vi "RPC Method queryserver_QueryServer_Register.vi"(8 "error in (no error)":errorcluster, 11 "OOP Server in":refnum<class "TestDataMarshal.lvclass">) -> (0 "error out":errorcluster, 3 "OOP Server out":refnum<class "TestDataMarshal.lvclass">)   [LabVIEW 2019, in "TestDataMarshal.lvlib" / "TestDataMarshal.lvclass"]
uses:
  TestDataMarshal.lvclass
  TestDataMarshal.lvclass/TestDataMarshal.ctl
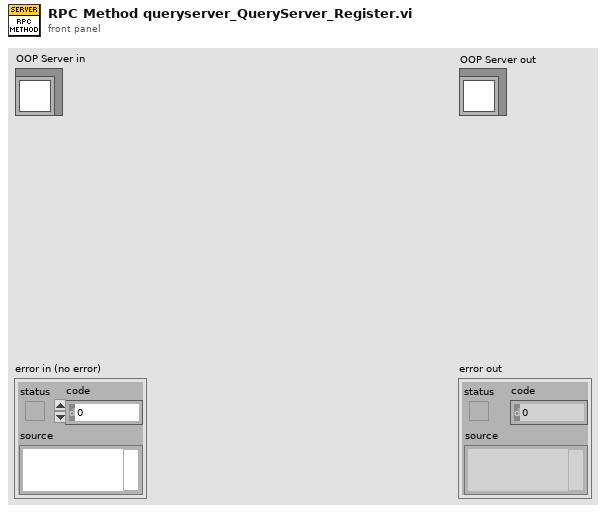
[diagram p1: front panel]
types:
  T1 = typedef "TestDataMarshal.lvlib/TestDataMarshal.lvclass/Server Internal UEs.ctl" = cluster{"queryserver_QueryServer_Invoke Internal UE":refnum<user-event>, "queryserver_QueryServer_Query Internal UE":refnum<user-event>, "queryserver_QueryServer_Register Internal UE":refnum<user-event>, "queryserver_QueryServer_TestDataTypes Internal UE":refnum<user-event>}
  T2 = typedef "TestDataMarshal.lvlib/TestDataMarshal.lvclass/Server gRPC UEs.ctl" = cluster{"queryserver_QueryServer_Invoke gRPC UE":refnum<user-event>, "queryserver_QueryServer_Query gRPC UE":refnum<user-event>, "queryserver_QueryServer_Register gRPC UE":refnum<user-event>, "queryserver_QueryServer_TestDataTypes gRPC UE":refnum<user-event>}
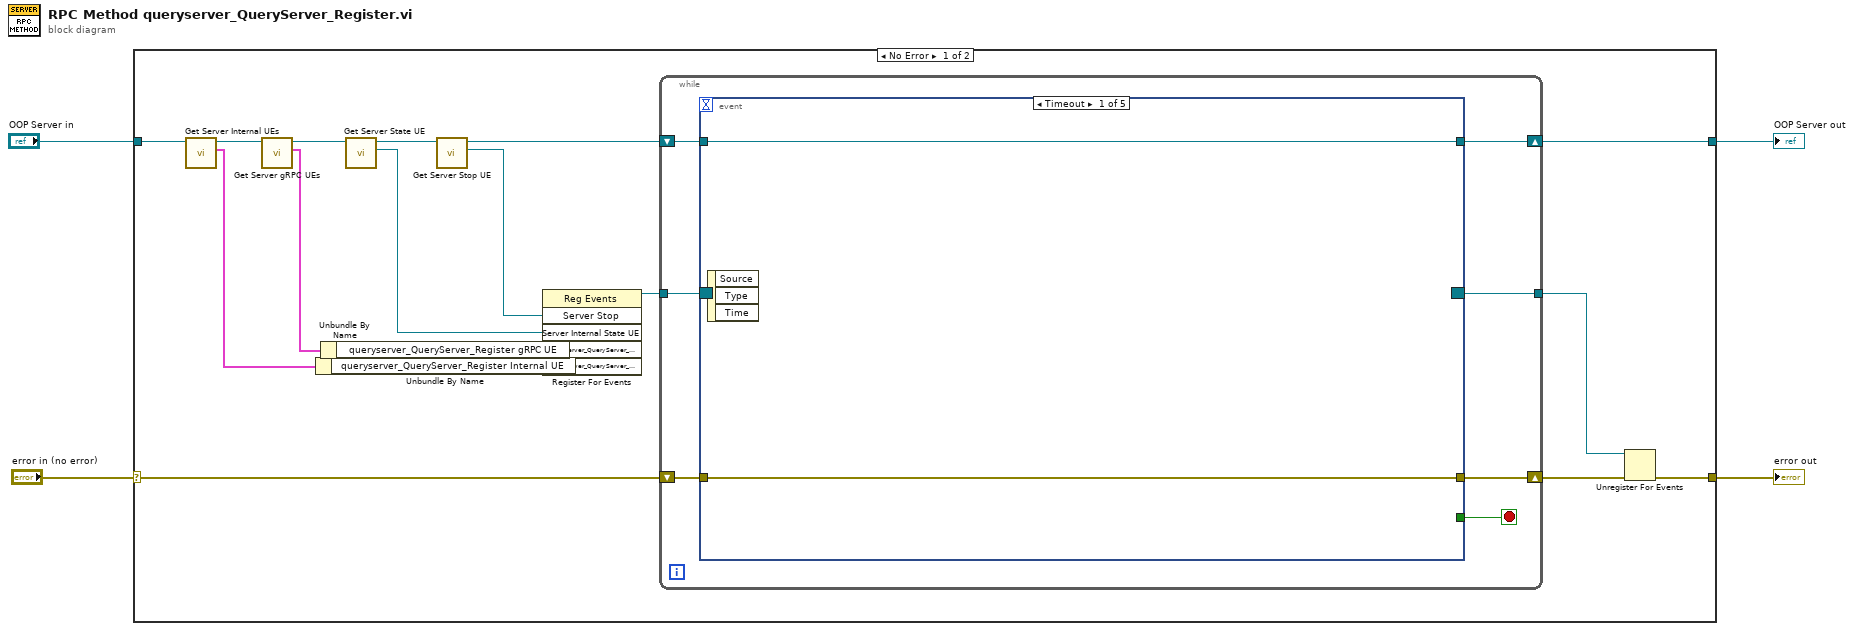
[diagram p0: block diagram]
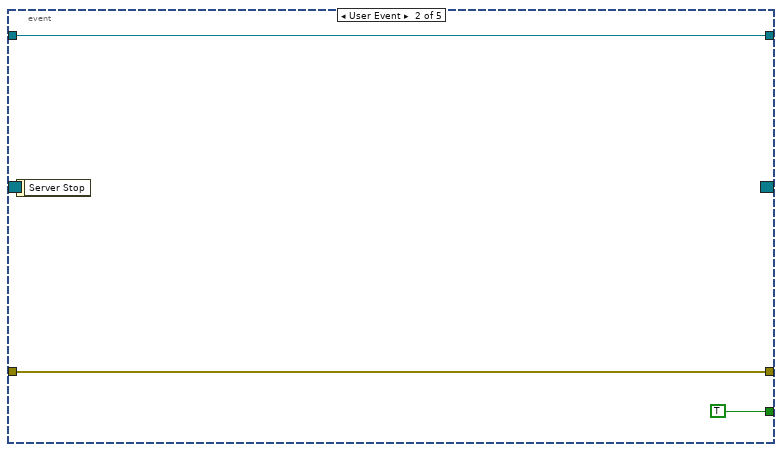
[diagram p2: hidden frame]
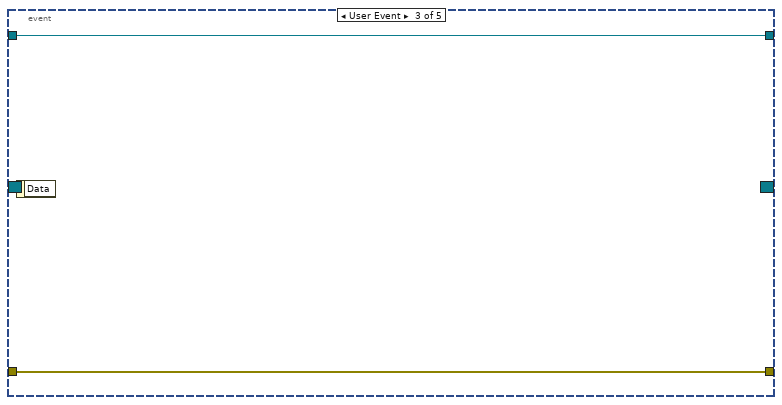
[diagram p3: hidden frame]
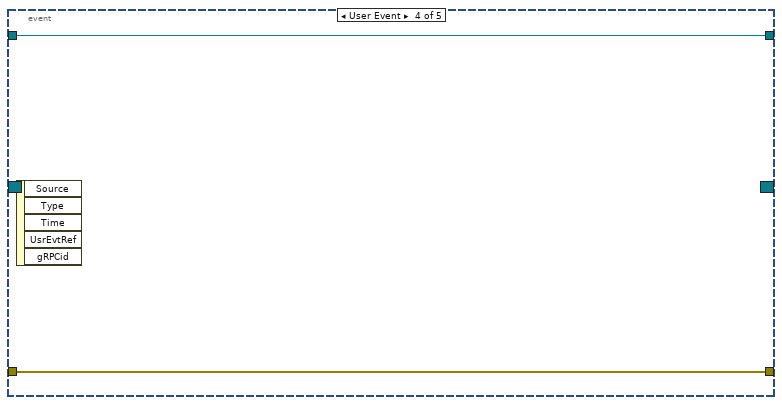
[diagram p4: hidden frame]
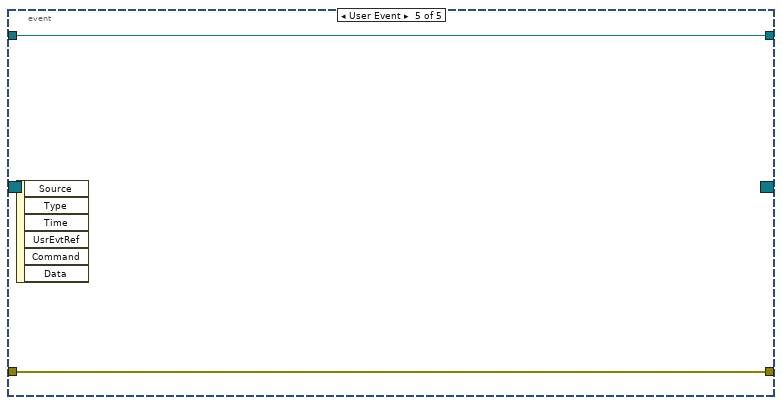
[diagram p5: hidden frame]
diagram:
  n1 = case shown="No Error" "error in (no error)" {
    selector: "error in (no error)" -> [w17 w41]
    tunnel: [w15 w41] -> w3
    tunnel: "OOP Server in" -> [w19 w40]
    tunnel: [w5 w40] -> w1
    frame No Error {
      n2 = call "Get Server Internal UEs.vi"("OOP Server in"=w19) -> ("Server Internal UEs"=w11:T1, "OOP Server out"=w18:refnum<class "TestDataMarshal.lvclass">)  [unwired: 9 in]
      n3 = call "Get Server gRPC UEs.vi"("OOP Server in"=w18) -> ("Server RPC Methods"=w13:T2, "OOP Server out"=w8:refnum<class "TestDataMarshal.lvclass">)  [unwired: 9 in]
      n4 = Unbundle By Name ("Unbundle Internal UE")(w11) -> ("queryserver_QueryServer_Register Internal UE"=w10:refnum<user-event>)
      n5 = Unbundle By Name ("Unbundle gRPC UE")(w13) -> ("queryserver_QueryServer_Register gRPC UE"=w12:refnum<user-event>)
      n6 = call "Get Server State UE.vi"("Template Server in"=w8) -> ("Server Internal State UE"=w6:refnum<user-event>, "Template Server out"=w7:refnum<class "TestDataMarshal.lvclass">)  [unwired: 9 in]
      n7 = call "Get Server Stop UE.vi"("OOP Server in"=w7) -> ("Server Stop"=w21:refnum<user-event>, "OOP Server out"=w9:refnum<class "TestDataMarshal.lvclass">)  [unwired: 9 in]
      n8 = register-events(w21, w6, w12, w10) -> (reference out=w20:refnum<event-registration>)  [unwired: 2 in, 1 out]
      n9 = while {
        tunnel: w20 -> [w28]
        tunnel: [w24] -> w14
        shift-right: [w25] -> w16
        shift-left: w17 -> [w26]
        shift-right: [w22] -> w5
        shift-left: w9 -> [w23]
        stop <- w27 stop-if-true
        n10 = event "RPC Method Event Structure" shown="[0] Timeout" {
          selector: w28 -> [_ _ _ _ _]
          dyn-events: [_ _ _ _ _] -> w24
          timeout: _ -> [_ _ _ _ _]
          tunnel: [_ TRUE _ _ _] -> w27
          tunnel: w26 -> [w30 w32 w35 w37 w39]
          tunnel: [w30 w32 w35 w37 w39] -> w25
          tunnel: w23 -> [w29 w31 w34 w36 w38]
          tunnel: [w29 w31 w34 w36 w38] -> w22
          event Timeout {
            n11 = event-data() -> ()  [unwired: 1 in, 3 out]
          }
          event User Event {
            n12 = event-data() -> ()  [unwired: 1 in, 1 out]
          }
          event User Event {
            n13 = event-data() -> ()  [unwired: 1 in, 1 out]
          }
          event User Event {
            n14 = event-data() -> ()  [unwired: 1 in, 5 out]
          }
          event User Event {
            n15 = event-data() -> ()  [unwired: 1 in, 6 out]
          }
        }
      }
      n16 = Unregister For Events(event registration refnum=w14, error in=w16) -> (error out=w15:errorcluster)
    }
    frame Error {
    }
  }
  "error out" <- w3
  "OOP Server out" <- w1
